vi "Write Interface Configs.vi"(8 "error in (no error)":errorcluster, 10 "Device Ref in":T2 format="%.0x", 11 "Refnum in":T1) -> (0 "error out":errorcluster, 2 "Item Ref out":T2 format="%.0x", 3 "Refnum out":T1)   [LabVIEW 2015, in "Modbus Master System Explorer.lvlib"]
uses:
  Modbus Master System Explorer.lvlib
  <vilib>/NI Veristand/Custom Device API/Custom Device Item Ref.ctl
  <vilib>/Utility/config.llb/Config Data RefNum.ctl
  <vilib>/Utility/config.llb/Write Key (String).vi
  <vilib>/Utility/config.llb/Write Key (U32).vi
  <vilib>/Utility/config.llb/NI_LVConfig.lvlib
  <vilib>/NI VeriStand/Custom Device API/Custom Device API.lvlib
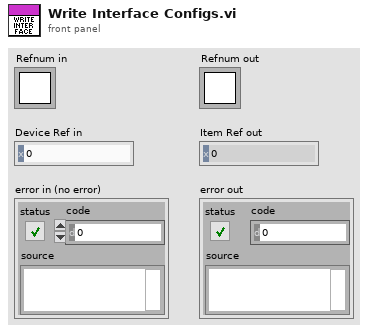
[diagram p1: front panel]
types:
  T1 = typedef "NI_LVConfig.lvlib/Config Data RefNum.ctl" = refnum<k1>
  T2 = typedef "Custom Device API.lvlib/Custom Device Item Ref.ctl" = u64
  T3 = typedef "Modbus Master Shared.lvlib/Interface Type.ctl" = enum16{"TCP Master", "Serial Master", "TCP Slave", "Serial Slave"}
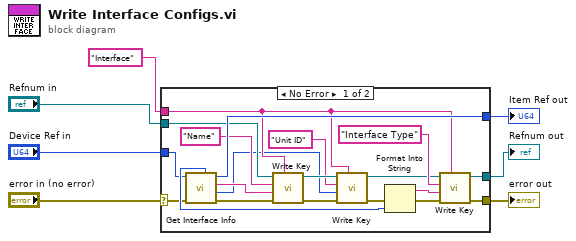
[diagram p0: block diagram]
diagram:
  n1 = case shown="No Error" "error in (no error)" {
    selector: "error in (no error)" -> [w16 w28]
    tunnel: [w23 w30] -> w7
    tunnel: [w22 w28] -> w6
    tunnel: [w21 w29] -> w5
    tunnel: "Interface" ("section") -> [w19 _]
    tunnel: "Device Ref in" -> [w15 w30]
    tunnel: "Refnum in" -> [w14 w29]
    frame No Error {
      n2 = call "Get Interface Info.vi"("error in (no error)"=w16, "Device Item Ref in"=w15) -> ("error out"=w17:errorcluster, "Unit ID"=w9:u16, "Name"=w12:string, "Item Ref out"=w23:T2, "Interface Type"=w26:T3)  [unwired: 4 in, 1 out]
      n3 = call-poly <vilib>:"Write Key.vi"("section"=w19, "error in (no error)"=w17, "value"=w12, "key"="Name", "refnum"=w14) -> ("error out"=w11:errorcluster, "refnum out"=w10:T1)  [unwired: 4 in, 1 out]
      n4 = call-poly <vilib>:"Write Key.vi"("section"=w19, "error in (no error)"=w11, "value"=w9, "key"="Unit ID", "refnum"=w10) -> ("error out"=w24:errorcluster, "refnum out"=w18:T1)  [unwired: 4 in, 1 out]
      n5 = Format Into String(error in=w24, w26) -> (resulting string=w27:string, error out=w25:errorcluster)  [unwired: 2 in]
      n6 = call-poly <vilib>:"Write Key.vi"("section"=w19, "error in (no error)"=w25, "value"=w27, "key"="Interface Type", "refnum"=w18) -> ("error out"=w22:errorcluster, "refnum out"=w21:T1)  [unwired: 4 in, 1 out]
    }
    frame Error {
    }
  }
  "Item Ref out" <- w7
  "error out" <- w6
  "Refnum out" <- w5
